vi "updateIndex.vi"(10 "index":string) -> (2 "new index":string)   [LabVIEW 2018]
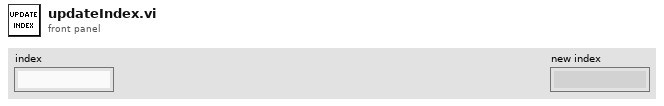
[diagram p1: front panel]
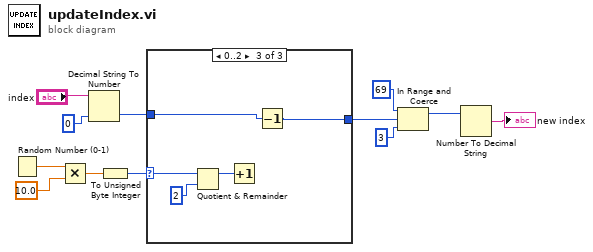
[diagram p0: block diagram]
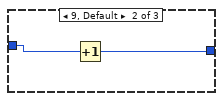
[diagram p3: hidden frame]
diagram:
  n1 = Random Number (0-1)() -> (number: 0 to 1=w10:dbl)
  n2 = Multiply(x=w10, y=10.0) -> (x*y=w8:dbl)
  n3 = Decimal String To Number(string="index", default (0L)=u8 0) -> (number=w6:u8)  [unwired: 1 in, 1 out]
  n4 = To Unsigned Byte Integer(number=w8) -> (unsigned 8bit integer=w7:u8)
  n5 = case shown="0..2" w7 {
    selector: w7 -> [_ _ w20]
    tunnel: w6 -> [w13 w15 w17]
    tunnel: [w13 w14 w16] -> w5
    frame 3..8 {
    }
    frame 9, Default {
      n6 = Increment(x=w15) -> (x+1=w14:u8)
    }
    frame 0..2 {
      n7 = Quotient & Remainder(x=w20, y=u8 2) -> (x-y*floor(x/y)=w18:u8)  [unwired: 1 out]
      n8 = Increment(x=w18) -> ()  [unwired: 1 out]
      n9 = Decrement(x=w17) -> (x-1=w16:u8)
    }
  }
  n10 = In Range and Coerce(upper limit=u8 69, x=w5, lower limit=u8 3) -> (coerced(x)=w1:u8)  [unwired: 1 out]
  n11 = Number To Decimal String(number=w1) -> (decimal integer string=→"new index":string)  [unwired: 1 in]
